vi "ConvStringIntoHex (SubVI).vi"(8 "Error In":errorcluster, 11 "String In":string) -> (0 "Error Out":errorcluster, 3 "Array Out":i64[](array[numeric]) format="%x")   [LabVIEW 2018]
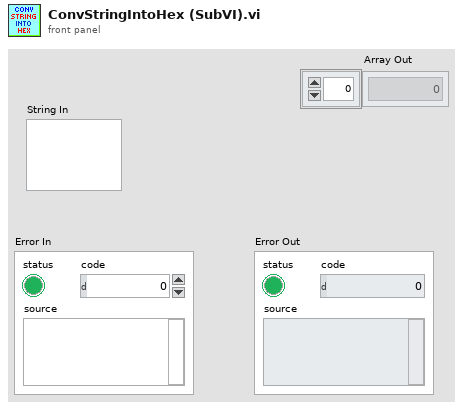
[diagram p1: front panel]
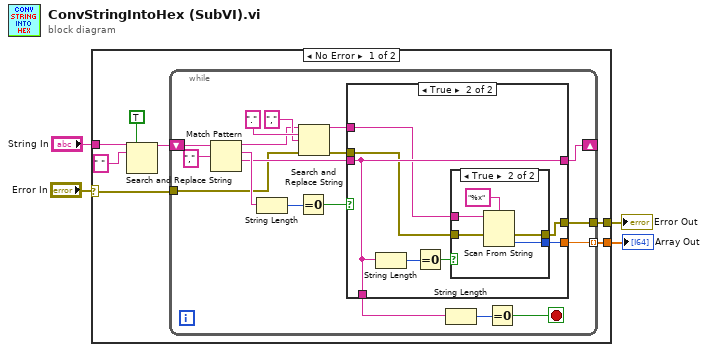
[diagram p0: block diagram]
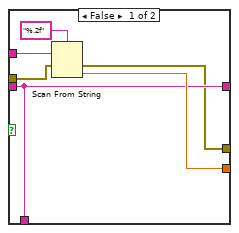
[diagram p2: hidden frame]
diagram:
  n1 = case shown="No Error" "Error In" {
    selector: "Error In" -> [w5 w49]
    tunnel: [w11 _] -> w4
    tunnel: "String In" -> [w8 _]
    tunnel: [w6 w49] -> w2
    frame No Error {
      n2 = Search and Replace String(replace all?=TRUE ("replace all? (F)"), input string=w8, search string=" ") -> (result string=w7:string)  [unwired: 5 in, 3 out]
      n3 = while {
        shift-right: [w25] -> _
        shift-left: w7 -> [w29]
        tunnel: [w21] -> w11 mode=indexing
        tunnel: w5 -> [w14]
        tunnel: [w12] -> w6
        stop <- w20 stop-if-true
        n4 = Match Pattern(string=w29, regular expression="," ("string")) -> (before substring=w15:string, match substring=w27:string, after substring=w24:string)  [unwired: 1 in, 1 out]
        n5 = String Length(string=w27) -> (length=w28:i32)
        n6 = Equal To 0?(x=w28) -> (x = 0?=w26:bool)
        n7 = Search and Replace String(input string=w15, search string=".", replace string="," ("replace string (\"\")"), error in=w14) -> (result string=w16:string, error out=w13:errorcluster)  [unwired: 4 in, 2 out]
        n8 = case shown="True" w26 {
          tunnel: [w33 w39] -> w25
          tunnel: w24 -> [w33 w39]
          tunnel: [w33 w39] -> w23
          tunnel: [w34 w40] -> w21
          tunnel: w16 -> [w32 w38]
          tunnel: w13 -> [w30 w37]
          tunnel: [w31 w36] -> w12
          frame False {
            n9 = Scan From String(format string="%.2f", input string=w32, error in=w30) -> (error out=w31:errorcluster, output 1=w34:dbl)  [unwired: 2 in, 2 out]
          }
          frame True {
            n10 = String Length(string=w39) -> (length=w41:i32)
            n11 = Equal To 0?(x=w41) -> (x = 0?=w42:bool)
            n12 = case shown="True" w42 {
              tunnel: [_ w48] -> w40
              tunnel: w38 -> [_ w47]
              tunnel: w37 -> [w43 w45]
              tunnel: [w43 w44] -> w36
              frame False {
              }
              frame True {
                n13 = Scan From String(format string="%x", input string=w47, error in=w45) -> (error out=w44:errorcluster, output 1=w48:u32)  [unwired: 2 in, 2 out]
              }
            }
          }
        }
        n14 = String Length(string=w23) -> (length=w22:i32)
        n15 = Equal To 0?(x=w22) -> (x = 0?=w20:bool)
      }
    }
    frame Error {
    }
  }
  "Array Out" <- w4
  "Error Out" <- w2
